vi "Time.vi"(4 "Value":timestamp) -> (1 "Constant":refnum<class "Const_Time.lvclass">)   [LabVIEW 2021, in "Const_Time.lvclass"]
uses:
  Const_Time.lvclass
  Const_Time.lvclass/Const_Time.ctl
  Properties/Write Value.vi
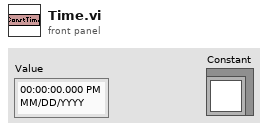
[diagram p1: front panel]
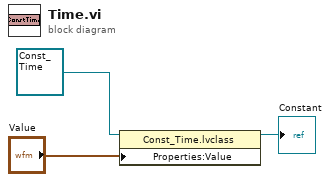
[diagram p0: block diagram]
diagram:
  n1 = property class="Const_Time.lvclass"(reference=refnum<class "Const_Time.lvclass"> refnum ("Constants.lvlib:Numeric.lvclass"), "Properties:Value"="Value") -> (reference out=→"Constant":refnum<class "Const_Time.lvclass">)  [unwired: 1 in, 1 out]
